vi "UDP Client.vi"(8 "Message":string, 10 "Port Number":u16, 11 "IP Address":string) -> ()   [LabVIEW 2016]
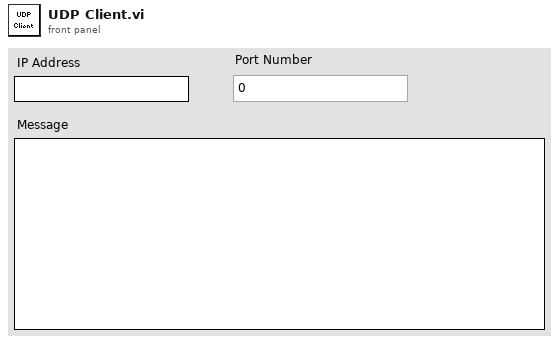
[diagram p1: front panel]
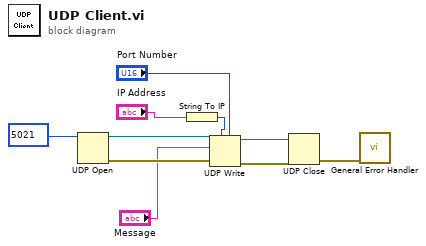
[diagram p0: block diagram]
diagram:
  n1 = UDP Open(11:u16 5021) -> (port=w8:refnum<k16>, 0:w7:errorcluster)  [unwired: 4 in, 1 out]
  n2 = String To IP(1:"IP Address") -> (0:w10:u32)
  n3 = UDP Write(address=w10, port or service name="Port Number", connection ID=w8, data in="Message", 8:w7) -> (error out=w4:errorcluster, 3:w5:refnum<k16>)  [unwired: 1 in]
  n4 = UDP Close(connection ID=w5, 8:w4) -> (error out=w3:errorcluster)  [unwired: 1 out]
  n5 = call <vilib>:"General Error Handler.vi"("error in (no error)"=w3) -> ()  [unwired: 10 in, 5 out]
